vi "Append Error Location.vi"(3 "error in (no error)":errorcluster, 4 "Chain Depth":i32) -> (5 "error out":errorcluster)   [LabVIEW 2021, in "CIFCoreCommon.lvlib"]
uses:
  CIFCoreCommon.lvlib
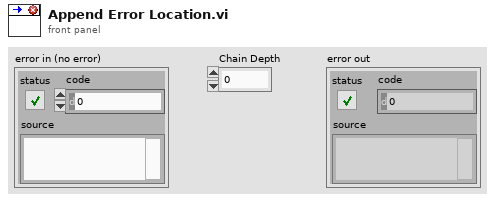
[diagram p1: front panel]
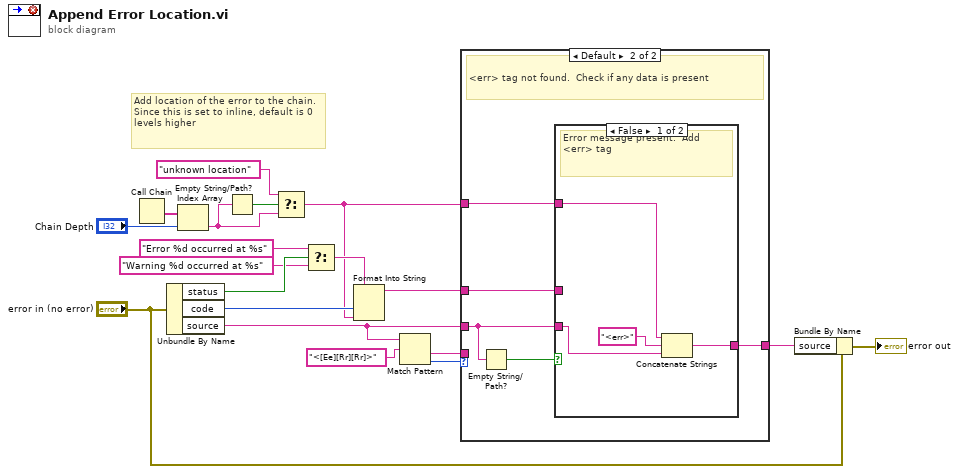
[diagram p0: block diagram]
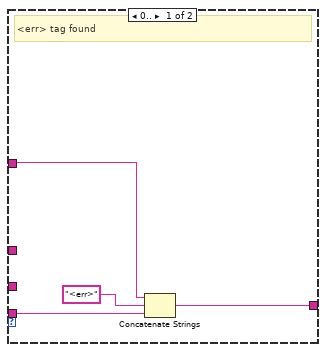
[diagram p2: hidden frame]
diagram:
  # "Add location of the error to the chain.  Since this is set to inline, default is 0 levels higher"
  n1 = Call Chain() -> (call chain=w18:string[])
  n2 = Unbundle By Name("error in (no error)") -> ("status"=w15:bool, "code"=w17:i32, "source"=w10:string)
  n3 = Index Array(array=w18, index="Chain Depth") -> (element=w3:string)
  n4 = Empty String/Path?(string/path=w3) -> (empty?=w4:bool)
  n5 = Select(t="unknown location", s=w4, f=w3) -> (s? t:f=w2:string)
  n6 = Select(t="Error %d occurred at %s" ("Error %d occurred at %s"), s=w15, f="Warning %d occurred at %s" ("Warning %d occurred at %s")) -> (s? t:f=w16:string)
  n7 = Format Into String(format string=w16, w17, w2) -> (resulting string=w9:string)  [unwired: 2 in, 1 out]
  n8 = Match Pattern(string=w10, regular expression="<[Ee][Rr][Rr]>" ("don't translate!")) -> (after substring=w8:string, offset past match=w11:i32)  [unwired: 1 in, 2 out]
  n9 = case shown="Default" w11 {
    tunnel: w10 -> [_ w27]
    tunnel: w9 -> [_ w24]
    tunnel: w2 -> [w20 w25]
    tunnel: w8 -> [w22 _]
    tunnel: [w21 w26] -> w6
    frame 0.. {
      # "<err> tag found"
      n10 = Concatenate Strings(w20, "<err>", w22) -> (w21:string)
    }
    frame Default {
      # "<err> tag not found.  Check if any data is present"
      n11 = Empty String/Path?(string/path=w27) -> (empty?=w28:bool)
      n12 = case shown="False" w28 {
        tunnel: w27 -> [w31 _]
        tunnel: [w30 w33] -> w26
        tunnel: w25 -> [w29 w33]
        tunnel: w24 -> [_ _]
        frame False {
          # "Error message present.  Add <err> tag"
          n13 = Concatenate Strings(w29, "<err>", w31) -> (w30:string)
        }
        frame True {
          # "No error message present.  Just add location information."
        }
      }
    }
  }
  n14 = Bundle By Name(cluster="error in (no error)", "source"=w6) -> (→"error out":errorcluster)
